vi "Check GU Number Arrange.vi"(8 "error in":errorcluster, 10 "Curr Cal Cfg In":T1, 11 "GU Arrange List":refnum<vi>) -> (0 "error out":errorcluster, 1 "Error Cell":T3(array[cluster]), 2 "Curr Cal Cfg Out":T1, 3 "GU Arrange List  Ref Out":refnum<vi>)   [LabVIEW 2020, in "GUCalibration2.lvlib"]
uses:
  GUCalibration2.lvlib
  Controls/Config Data Type.ctl
  Controls/GU Arrange Check Rule.ctl
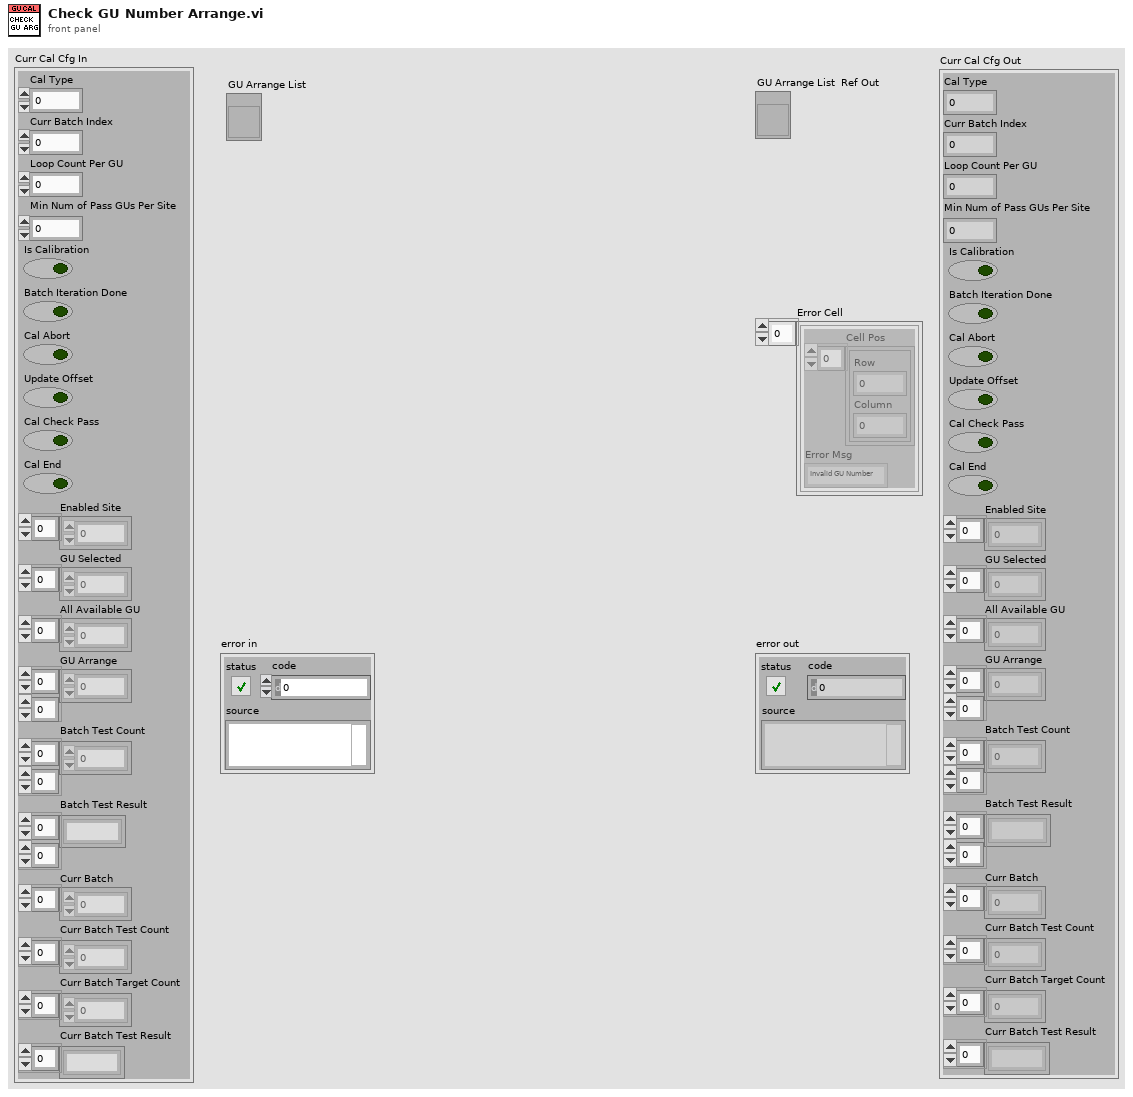
[diagram p1: front panel]
types:
  T1 = typedef "GUCalibration2.lvlib/Config Data Type.ctl" = cluster{"Cal Type":i32, "Curr Batch Index":i32, "Loop Count Per GU":i32, "Min Num of Pass GUs Per Site":i32, "Is Calibration":bool, "Batch Iteration Done":bool, "Cal Abort":bool, "Update Offset":bool, "Cal Check Pass":bool, "Cal End":bool, "Enabled Site":i32[], "GU Selected":i32[], "All Available GU":i32[], "GU Arrange":i32[][], "Batch Test Count":i32[][], "Batch Test Result":string[][], "Curr Batch":i32[], "Curr Batch Test Count":i32[], "Curr Batch Target Count":i32[], "Curr Batch Test Result":string[]}
  T2 = typedef "GUCalibration2.lvlib/GU Arrange Check Rule.ctl" = enum16{"Invalid GU Number", "GU Number Conflict"}
  T3 = cluster{"Cell Pos":cluster{"Row":i32, "Column":i32}[], "Error Msg":T2}[]
  T4 = cluster{"Cell Pos":cluster{"Row":i32, "Column":i32}[], "Enum":T2}[]
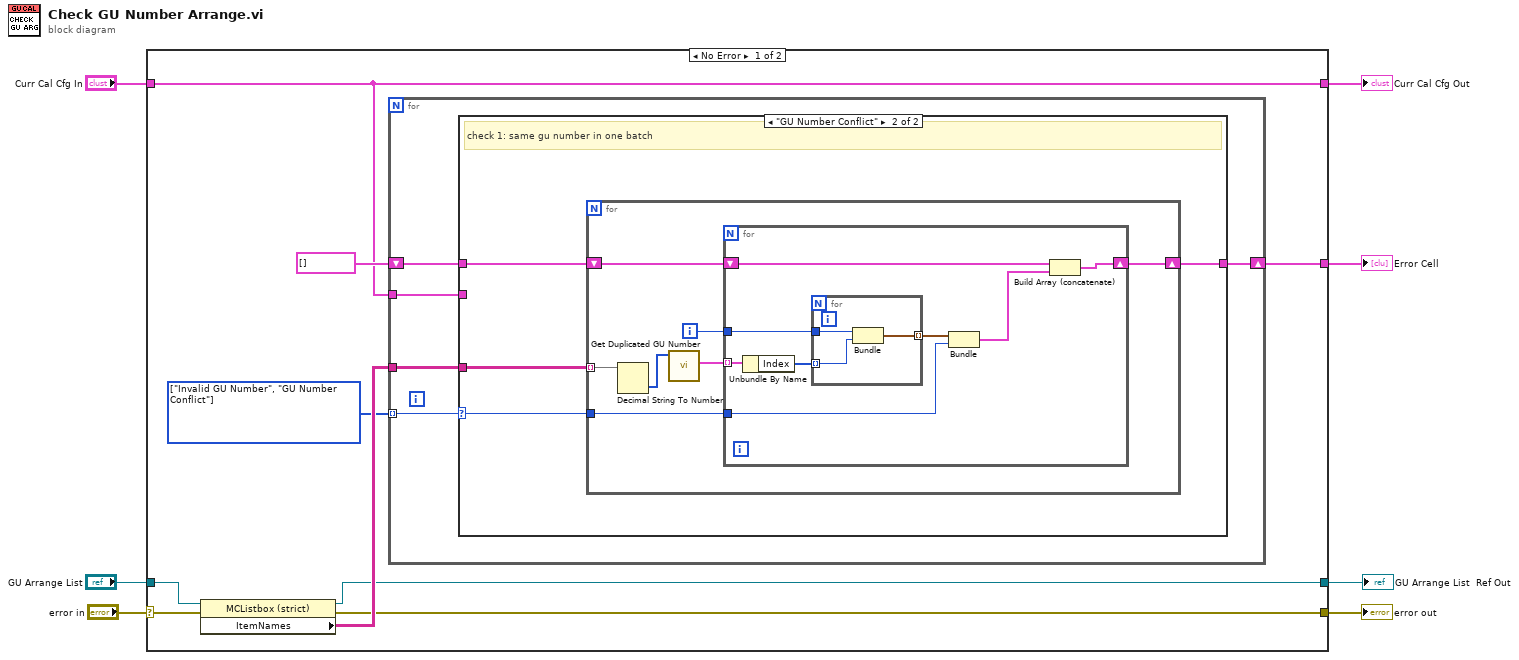
[diagram p0: block diagram]
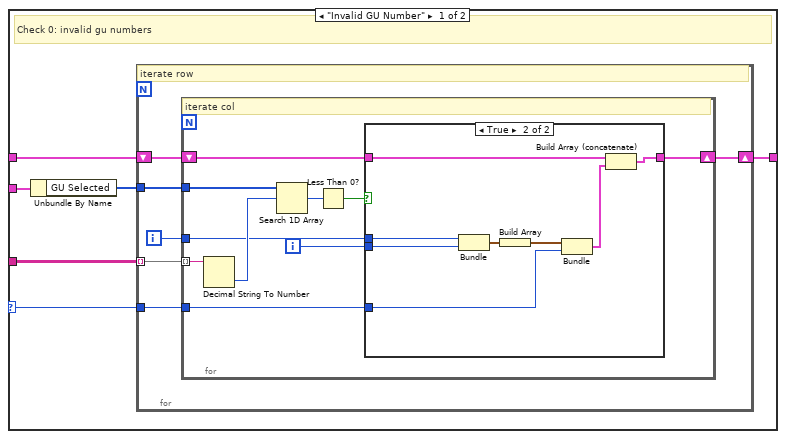
[diagram p2: hidden frame]
diagram:
  n1 = case shown="No Error" "error in" {
    selector: "error in" -> [w9 w76]
    tunnel: "GU Arrange List" -> [w16 w75]
    tunnel: "Curr Cal Cfg In" -> [w10 w77]
    tunnel: [w12 w76] -> w5
    tunnel: [w11 _] -> w4
    tunnel: [w10 w77] -> w2
    tunnel: [w8 w75] -> w1
    frame No Error {
      w13 = T2[] [enum."Invalid GU Number", enum."GU Number Conflict"] items=["Invalid GU Number", "GU Number Conflict"]
      n2 = property class="MCListbox (strict)"(reference=w16, error in=w9) -> (reference out=w8:refnum<vi>, error out=w12:errorcluster, "ItemNames"=w15:string[][])
      n3 = for {
        tunnel: w15 -> [w21]
        tunnel: w10 -> [w20]
        shift-right: [w18] -> w11
        shift-left: T3 [] ("Array") -> [w19]
        tunnel: w13 -> [w17] mode=indexing
        n4 = case shown="\"GU Number Conflict\"" w17 {
          selector: w17 -> [w22 w53]
          tunnel: w21 -> [w27 w56]
          tunnel: w20 -> [w26 _]
          tunnel: w19 -> [w24 w55]
          tunnel: [w23 w54] -> w18
          frame "Invalid GU Number" {
            # "Check 0: invalid gu numbers"
            n5 = Unbundle By Name(w26) -> ("GU Selected"=w25:i32[])
            n6 = for {
              tunnel: w27 -> [w33] mode=indexing
              tunnel: w25 -> [w32]
              shift-right: [w29] -> w23
              shift-left: w24 -> [w31]
              tunnel: w22 -> [w28]
              i -> [w30]
              # "iterate row"
              n7 = for {
                tunnel: w33 -> [w43] mode=indexing
                tunnel: w32 -> [w42]
                shift-right: [w36] -> w29
                shift-left: w31 -> [w39]
                tunnel: w30 -> [w38]
                tunnel: w28 -> [w34]
                i -> [w37]
                # "iterate col"
                n8 = Decimal String To Number(string=w43) -> (number=w41:i32)  [unwired: 2 in, 1 out]
                n9 = Search 1D Array(1D array=w42, element=w41) -> (index of element=w40:i32)  [unwired: 1 in]
                n10 = Less Than 0?(x=w40) -> (x < 0?=w35:bool)
                n11 = case shown="True" w35 {
                  tunnel: w39 -> [w44 w52]
                  tunnel: w38 -> [_ w50]
                  tunnel: w37 -> [_ w49]
                  tunnel: [w44 w46] -> w36
                  tunnel: w34 -> [_ w45]
                  frame False {
                  }
                  frame True {
                    n12 = Bundle(w50, w49) -> (w48:cluster{i32, i32})  [unwired: 1 in]
                    n13 = Build Array(w48) -> (w51:cluster{i32, i32}[])
                    n14 = Bundle(w51, "Enum"=w45) -> (w47:cluster{cluster{i32, i32}[], "Enum":T2})  [unwired: 1 in]
                    n15 = Build Array (concatenate)(w52, w47) -> (w46:T4)
                  }
                }
              }
            }
          }
          frame "GU Number Conflict" {
            # "check 1: same gu number in one batch"
            n16 = for {
              tunnel: w56 -> [w63] mode=indexing
              shift-right: [w60] -> w54
              shift-left: w55 -> [w61]
              tunnel: w53 -> [w57]
              i -> [w62]
              n17 = Decimal String To Number(string=w63) -> (number=w59:i32[])  [unwired: 2 in, 1 out]
              n18 = call "Get Duplicated GU Number.vi"("GU Numbers"=w59) -> ("Repeated GU"=w58:cluster{"GU Number":i32, "Index":i32[]}[])  [unwired: 9 in, 1 out]
              n19 = for {
                tunnel: w58 -> [w71] mode=indexing
                tunnel: w62 -> [w67]
                shift-right: [w69] -> w60
                shift-left: w61 -> [w70]
                tunnel: w57 -> [w64]
                n20 = Unbundle By Name(w71) -> ("Index"=w68:i32[])
                n21 = for {
                  tunnel: w67 -> [w74]
                  tunnel: w68 -> [w73] mode=indexing
                  tunnel: [w72] -> w66 mode=indexing
                  n22 = Bundle(w74, w73) -> (w72:cluster{i32, i32})  [unwired: 1 in]
                }
                n23 = Bundle(w66, "Enum"=w64) -> (w65:cluster{cluster{i32, i32}[], "Enum":T2})  [unwired: 1 in]
                n24 = Build Array (concatenate)(w70, w65) -> (w69:T4)
              }
            }
          }
        }
      }
    }
    frame Error {
    }
  }
  "error out" <- w5
  "Error Cell" <- w4
  "Curr Cal Cfg Out" <- w2
  "GU Arrange List  Ref Out" <- w1
